vi "At Minimum.vi"() -> ()   [LabVIEW 2017, in "Assertions.Tests.lvlib" / "Assert Not In Range.lvlib"]
uses:
  Assert Not In Range.lvlib
  fbabce95-ee89-44c7-8094-e68d7d4e1db2.vi
  src/Transparent Assertions/Constraints/Logical And/Logical And.lvclass
  C:/Users/pasca/Projects/Home/TransparentAssertions/src/Transparent Assertions/Constraints/Binary Operator/Binary Operator.lvclass
  C:/Users/pasca/Projects/Home/TransparentAssertions/src/Transparent Assertions/Constraints/Constraint/Constraint.lvclass
  src/Transparent Assertions/Constraints/Logical Or/Logical Or.lvclass
  src/Transparent Assertions/Constraints/Is Less Than/Is Less Than.lvclass
  src/Transparent Assertions/Constraints/IsEqual/IsEqual.lvclass
  src/Transparent Assertions/Constraints/Is Greater Than/Is Greater Than.lvclass
  src/Transparent Assertions/Constraints/IsEqual/Create.vi
  src/Transparent Assertions/Constraints/Is Less Than/Create.vi
  src/Transparent Assertions/Constraints/Binary Operator/Create.vi
  src/Transparent Assertions/Constraints/Is Greater Than/Create.vi
  src/Transparent Assertions/Constraints/LogicalNot/LogicalNot.lvclass
  src/Transparent Assertions/Constraints/UnaryOperator/UnaryOperator.lvclass
  src/Transparent Assertions/Assertions/Assertions.lvlib
panel:
  out "error out":errorcluster
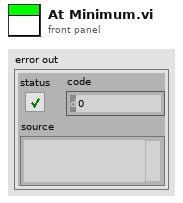
[diagram p1: front panel]
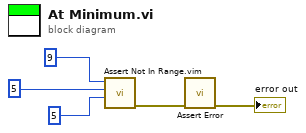
[diagram p0: block diagram]
diagram:
  n1 = call "Assert Not In Range.vim"("Minimum"=5, "Actual"=5, "Maximum"=9) -> ("error out"=w1:errorcluster)  [unwired: 8 in]
  n2 = call "Assert Error.vi"("error in (no error)"=w1) -> ("error out"=→"error out":errorcluster)  [unwired: 10 in]
